vi "GoPro Init.vi"() -> (0 "error out":errorcluster, 3 "Gopro DevRef":T1)   [LabVIEW 2015]
uses:
  GoPro DevRef.ctl
  <vilib>/httpClient/ClientHandle.ctl
  <vilib>/httpClient/LabVIEWHTTPClient.lvlib
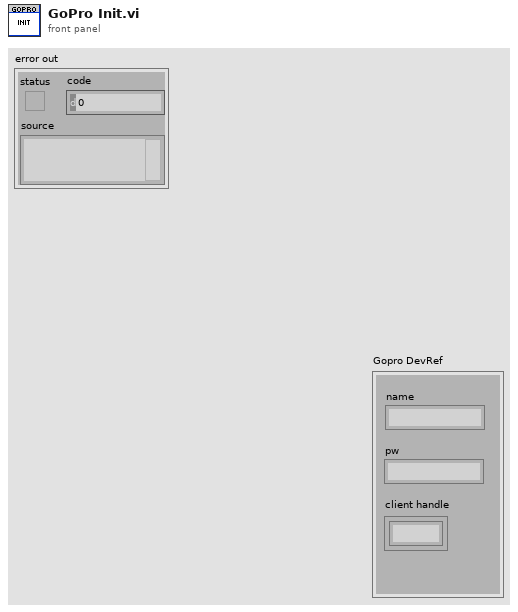
[diagram p1: front panel]
types:
  T1 = typedef "GoPro DevRef.ctl" = cluster{"name":string, "pw":string, "client handle":T2}
  T2 = typedef "LabVIEWHTTPClient.lvlib/ClientHandle.ctl" = refnum<k1>
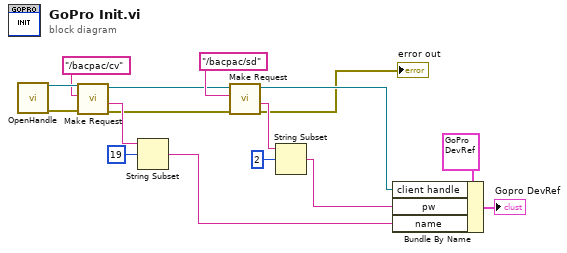
[diagram p0: block diagram]
diagram:
  n1 = call <vilib>:"OpenHandle.vi"() -> ("client handle out"=w16:T2, "error out"=w3:errorcluster)  [unwired: 14 in]
  n2 = call "Make Request.vi"("error in (no error)"=w3, "url"="/bacpac/cv", "Refnum in"=w16) -> ("error out"=w2:errorcluster, "body"=w14:string, "client handle out"=w11:T2)  [unwired: 5 in, 1 out]
  n3 = String Subset(string=w14, offset (0)=19) -> (substring=w6:string)  [unwired: 1 in]
  n4 = call "Make Request.vi"("error in (no error)"=w2, "url"="/bacpac/sd", "Refnum in"=w11) -> ("error out"=→"error out":errorcluster, "body"=w9:string, "client handle out"=w4:T2)  [unwired: 5 in, 1 out]
  n5 = String Subset(string=w9, offset (0)=2) -> (substring=w7:string)  [unwired: 1 in]
  n6 = Bundle By Name(cluster=T1 {"name"="JamsGoPro", "pw"="yoloswag666", "client handle"=refnum} ("Gopro DevRef"), "client handle"=w4, "pw"=w7, "name"=w6) -> (→"Gopro DevRef":T1)
